vi "Get Finger Positions.vi"(8 "error in (no error)":errorcluster, 11 "MF3 in":refnum<class "MF3.lvclass">) -> (0 "error out":errorcluster, 1 "Triangle Centroid Pose":T1, 2 "Finger Positions":T4, 3 "MF3 out":refnum<class "MF3.lvclass">)   [LabVIEW 2013, in "MF3.lvclass"]
uses:
  MF3.lvclass
  controls/Vector3D Fingers.ctl
  labview_ros/geometry_msgs/Pose.ctl
  labview_ros/geometry_msgs/Point.ctl
  labview_ros/geometry_msgs/Quaternion.ctl
  MF3.lvclass/MF3.ctl
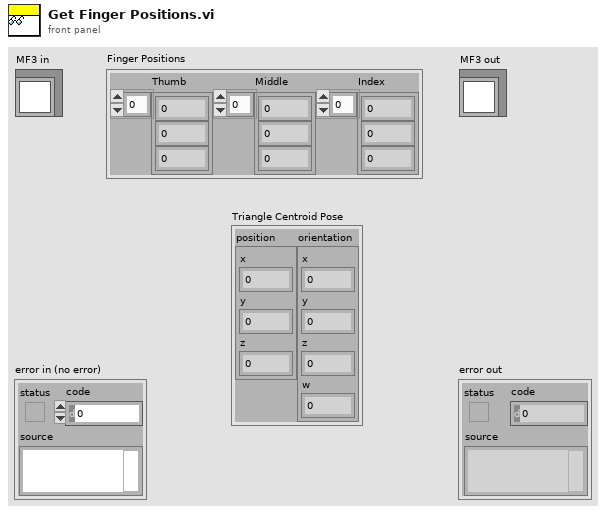
[diagram p1: front panel]
types:
  T1 = typedef "Pose.ctl" = cluster{"position":T2, "orientation":T3}
  T2 = typedef "Point.ctl" = cluster{"x":dbl, "y":dbl, "z":dbl}
  T3 = typedef "Quaternion.ctl" = cluster{"x":dbl, "y":dbl, "z":dbl, "w":dbl}
  T4 = typedef "Vector3D Fingers.ctl" = cluster{"Thumb":dbl[], "Middle":dbl[], "Index":dbl[]}
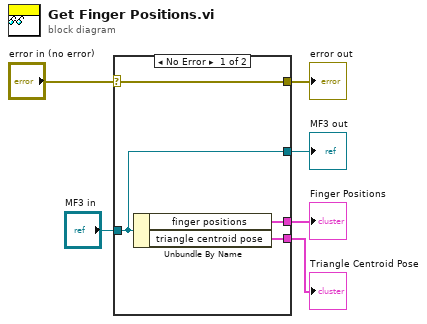
[diagram p0: block diagram]
diagram:
  n1 = case shown="No Error" "error in (no error)" {
    selector: "error in (no error)" -> [w10 w11]
    tunnel: [w10 w11] -> w5
    tunnel: [w9 w12] -> w3
    tunnel: "MF3 in" -> [w9 w12]
    tunnel: [w8 _] -> w2
    tunnel: [w7 _] -> w1
    frame No Error {
      n2 = Unbundle By Name(w9) -> ("finger positions"=w8:T4, "triangle centroid pose"=w7:T1)
    }
    frame Error {
    }
  }
  "error out" <- w5
  "MF3 out" <- w3
  "Finger Positions" <- w2
  "Triangle Centroid Pose" <- w1
